vi "random-neg-pos.vi"() -> (0 "out":dbl)   [LabVIEW 2015]
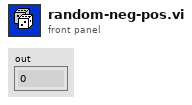
[diagram p1: front panel]
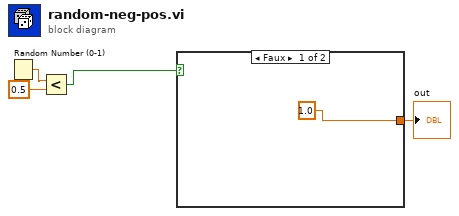
[diagram p0: block diagram]
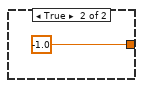
[diagram p2: hidden frame]
diagram:
  n1 = Random Number (0-1)() -> (number: 0 to 1=w2:dbl)
  n2 = Less?(x=w2, y=0.5) -> (x < y?=w3:bool)
  n3 = case shown="Faux" w3 {
    tunnel: [1.0 -1.0] -> w4
    frame False {
    }
    frame True {
    }
  }
  "out" <- w4
